vi "3D-IP地址转换.vi"(5 "IP地址":string="192.168.1.25") -> (0 "数组":string[](array[string]), 4 "IP数组":i32[](array[numeric]))   [LabVIEW 2015]
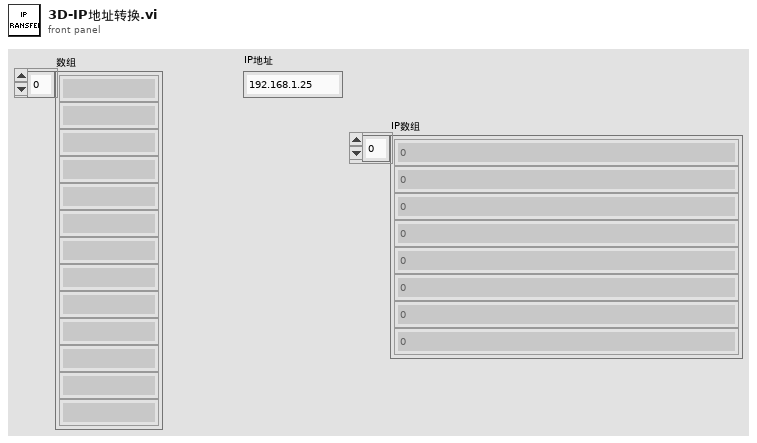
[diagram p1: front panel]
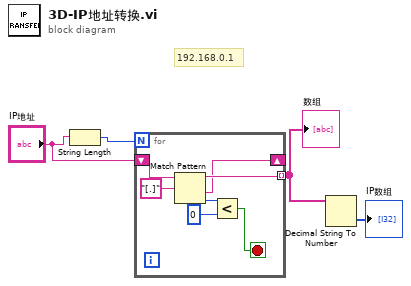
[diagram p0: block diagram]
diagram:
  # "192.168.0.1"
  n1 = String Length(string="IP地址") -> (length=w3:i32)
  n2 = for {
    N: w3 -> [_]
    tunnel: [w9] -> w2 mode=indexing
    shift-right: [w8] -> _
    shift-left: "IP地址" -> [w11]
    stop <- w5 stop-if-true
    n3 = Match Pattern(string=w11, regular expression="[.]" ("正则表达式")) -> (before substring=w9:string, after substring=w8:string, offset past match=w7:i32)  [unwired: 1 in, 1 out]
    n4 = Less?(x=w7, y=0) -> (x < y?=w5:bool)
  }
  "数组" <- w2
  n5 = Decimal String To Number(string=w2) -> (number=→"IP数组":i32[])  [unwired: 2 in, 1 out]
